vi "DispenseDosage_SubVI.vi"(9 "Numeric 2":i32, 10 "Numeric":i32, 11 "BrickReference in":T1) -> (3 "BrickReference out":T1)   [LabVIEW 2016]
uses:
  <vilib>/NXT/Subs/LVHSConnector.ctl
  <vilib>/NXT/LegoClasses/BrickReference/BrickReference.lvclass
  <vilib>/NXT/Block Support/NXT_OutputPort.ctl
  <vilib>/NXT/NXTIO Xnodes/NXTIONodeSubVIs/NXTMotorRunDistance.vi
  <vilib>/NXT/Dual Mode Library/Waits/Wait_Num.vi
  <vilib>/NXT/NXTIO Xnodes/AddressXNode/NXTIOAddress.xnode
  <vilib>/NXT/NXTIO Xnodes/NXTIOXNode/NXTIO.xnode
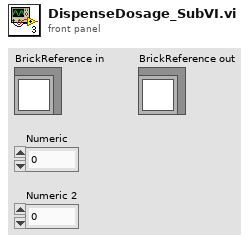
[diagram p1: front panel]
types:
  T1 = typedef "LVHSConnector.ctl" = refnum<class "BrickReference.lvclass">
  T2 = typedef "NXT_OutputPort.ctl" = u8
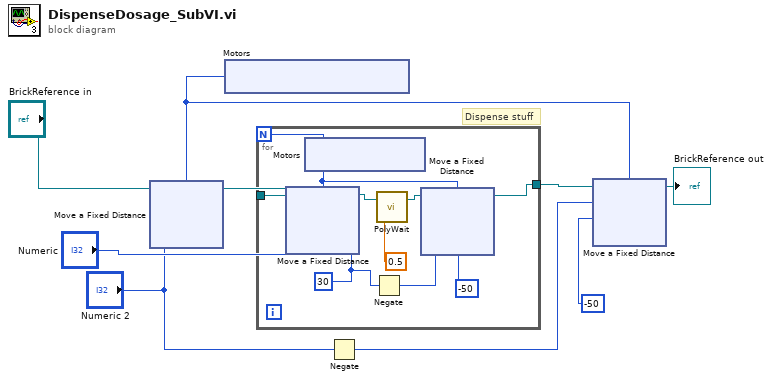
[diagram p0: block diagram]
diagram:
  # "Dispense stuff"
  n1 = xnode "Motors"() -> ("Motor"=w3:T2)
  n2 = xnode "Move a Fixed Distance"("Distance 1"="Numeric 2", "Motors"=w3, "NXT/EV3"="BrickReference in") -> ("NXT/EV3"=w7:T1)  [unwired: 1 in]
  n3 = for {
    N: "Numeric" -> [_]
    tunnel: w7 -> [w18]
    tunnel: [w11] -> w8
    w17 = 30
    n4 = xnode "Motors"() -> ("Motor"=w10:T2)
    n5 = xnode "Move a Fixed Distance"("Distance 1"=w17, "Motors"=w10, "NXT/EV3"=w18) -> ("NXT/EV3"=w13:T1)  [unwired: 1 in]
    n6 = Negate(x=w17) -> (-x=w15:i32)
    n7 = call-poly <vilib>:"PolyWait.vi"("Time (1 sec)"=sgl 0.5, "NXT/EV3"=w13) -> ("NXT/EV3"=w12:T1)  [unwired: 2 in]
    n8 = xnode "Move a Fixed Distance"("Speed 1"=i8 -50, "Distance 1"=w15, "Motors"=w10, "NXT/EV3"=w12) -> ("NXT/EV3"=w11:T1)
  }
  n9 = Negate(x="Numeric 2") -> (-x=w4:i32)
  n10 = xnode "Move a Fixed Distance"("Speed 1"=i8 -50, "Distance 1"=w4, "Motors"=w3, "NXT/EV3"=w8) -> ("NXT/EV3"=→"BrickReference out":T1)
